vi "Grapher_Create.vi"(0 "reference in":refnum<class "Grapher.lvclass">, 1 "Indicator Refs":T1, 2 "Update Rate (ms)":i32=50, 3 "Graph Queue":refnum<queue>, 4 "HPS17K Refs":refnum<class "HPS-17000.lvclass">[](array[class]), 5 "Error In":errorcluster) -> (14 "reference out":refnum<class "Grapher.lvclass">, 19 "Error Out":errorcluster)   [LabVIEW 2023, in "Grapher.lvclass"]
uses:
  Grapher.lvclass
  Types/Indicators.ctl
  <vilib>/HPS-17000/MStream_grpc_CyclerMeasurement.ctl
  <instrlib>/HPS-17000/HPS-17000.lvclass
  Grapher.lvclass/Grapher.ctl
  <vilib>/HPS-17000/NI_BC_client.lvlib
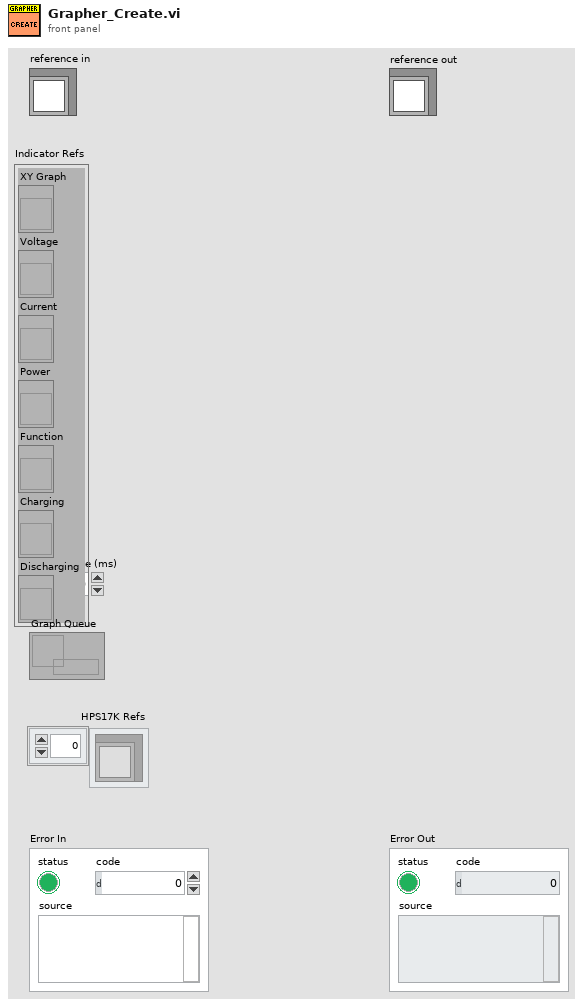
[diagram p1: front panel]
types:
  T1 = typedef "Indicators.ctl" = cluster{"XY Graph":refnum<vi>, "Voltage":refnum<vi>, "Current":refnum<vi>, "Power":refnum<vi>, "Function":refnum<vi>, "Charging":refnum<vi>, "Discharging":refnum<vi>}
  T2 = typedef "Grapher.lvclass/ObjectAttributes.ctl" = cluster{"Indicator Refs":T1, "Update Rate (ms)":i32, "Graph Queue":refnum<queue>, "HPS17K Refs":refnum<class "HPS-17000.lvclass">[]}
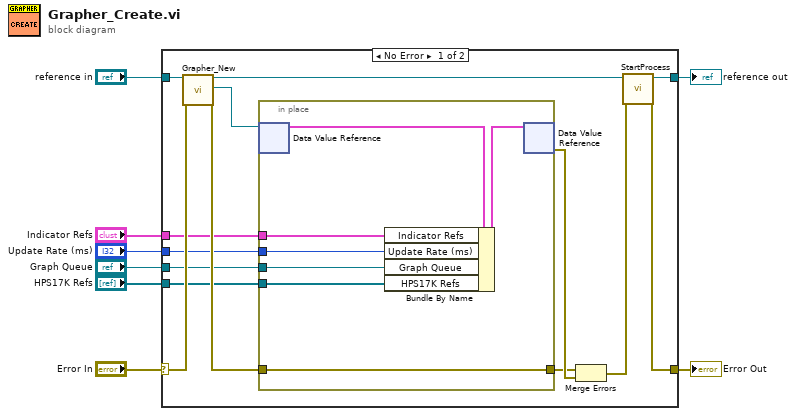
[diagram p0: block diagram]
diagram:
  n1 = case shown="No Error" "Error In" {
    selector: "Error In" -> [w21 w31]
    tunnel: [w13 w31] -> w7
    tunnel: "reference in" -> [w22 w30]
    tunnel: [w15 w30] -> w5
    tunnel: "Indicator Refs" -> [w12 _]
    tunnel: "Update Rate (ms)" -> [w11 _]
    tunnel: "Graph Queue" -> [w10 _]
    tunnel: "HPS17K Refs" -> [w9 _]
    frame No Error {
      n2 = call "Grapher_New.vi"("reference in"=w22, "Error In"=w21) -> ("reference out"=w16:refnum<class "Grapher.lvclass">, "DVRRefOut"=w19:refnum<data-value>, "Error Out"=w18:errorcluster)  [unwired: 14 in, 1 out]
      n3 = in-place {
        in-place-border: w18 -> [w27]
        in-place-border: [w27] -> w17
        in-place-border: w12 -> [w26]
        in-place-border: w11 -> [w25]
        in-place-border: w10 -> [w24]
        in-place-border: w9 -> [w23]
        n4 = in-place-dvr #1(w19) -> (w28:T2)  [unwired: 1 out]
        n5 = Bundle By Name(cluster=w28, "Indicator Refs"=w26, "Update Rate (ms)"=w25, "Graph Queue"=w24, "HPS17K Refs"=w23) -> (w29:T2)
        n6 = in-place-dvr #1(w29) -> (w20:errorcluster)  [unwired: 1 out]
      }
      n7 = Merge Errors(w17, w20) -> (w14:errorcluster)
      n8 = call "StartProcess.vi"("reference in"=w16, "Error In"=w14) -> ("reference out"=w15:refnum<class "Grapher.lvclass">, "Error Out"=w13:errorcluster)  [unwired: 14 in, 2 out]
    }
    frame Error {
      # "VI-TechBaseTemplate_Simple_6x8x6"
    }
  }
  "Error Out" <- w7
  "reference out" <- w5
